vi "Global_ACT Write_Data Out.vi"() -> ()   [LabVIEW 2017, in "Lift.lvlib"]
uses:
  Lift.lvlib
  CLUSTER_ACT_Lift Output.ctl
  _SHARE ALL/RoboRio Share All/SRX Share All/TypeDefs SRX/Cluster_SRX_General Data.ctl
  _SHARE ALL/RoboRio Share All/SRX Share All/TypeDefs SRX/Cluster_SRX_Common Runtime Data.ctl
  _SHARE ALL/RoboRio Share All/SRX Share All/TypeDefs SRX/Cluster_SRX_Error Calculations.ctl
  _SHARE ALL/RoboRio Share All/SRX Share All/TypeDefs SRX/Cluster_SRX_Voltage Out Data.ctl
  _SHARE ALL/RoboRio Share All/SRX Share All/TypeDefs SRX/Cluster_SRX_Sensor Out Data.ctl
  _SHARE ALL/RoboRio Share All/SRX Share All/TypeDefs SRX/Cluster_SRX_Sensor Quad Data.ctl
  _SHARE ALL/RoboRio Share All/SRX Share All/TypeDefs SRX/Cluster_SRX_Analog In Data.ctl
  _SHARE ALL/RoboRio Share All/SRX Share All/TypeDefs SRX/Cluster_SRX_PWM Sensor Data.ctl
  _SHARE ALL/RoboRio Share All/SRX Share All/TypeDefs SRX/Cluster_SRX_F and R Limit Indicators.ctl
panel:
  in  "Lift_ACT_Rotate_Output":T1 {"Common Runtime Data Out"."Temp" format="%.1f"; "Common Runtime Data Out"."Voltage"."Bus" format="%.3f"; "Common Runtime Data Out"."Voltage"."Output" format="%.3f"; "Common Runtime Data Out"."Voltage"."Percent" format="%.3f"; "Common Runtime Data Out"."Current" format="%.2f"}
  in  "Lift_ACT_Telescope_Output":T1 {"Common Runtime Data Out"."Temp" format="%.1f"; "Common Runtime Data Out"."Voltage"."Bus" format="%.3f"; "Common Runtime Data Out"."Voltage"."Output" format="%.3f"; "Common Runtime Data Out"."Voltage"."Percent" format="%.3f"; "Common Runtime Data Out"."Current" format="%.2f"}
  in  "Lift_ACT_Claw_Rotation_Output":T1 {"Common Runtime Data Out"."Temp" format="%.1f"; "Common Runtime Data Out"."Voltage"."Bus" format="%.3f"; "Common Runtime Data Out"."Voltage"."Output" format="%.3f"; "Common Runtime Data Out"."Voltage"."Percent" format="%.3f"; "Common Runtime Data Out"."Current" format="%.2f"}
  # "The Names of the Data items in the Global Variable MUST describe who the Single Writer is\nNaming Convention of all Data Items is:   \nLib Name_Loop Name (SM or SEN or ACT)_Data Name\nExamples:\nDrive_ACT_X axis\nGameController_SEN_JoystickLeft\nHopper_SM_AgitatorSpeed"
  # "C"
  # "Units"
  # "C"
  # "Units"
  # "C"
  # "Units"
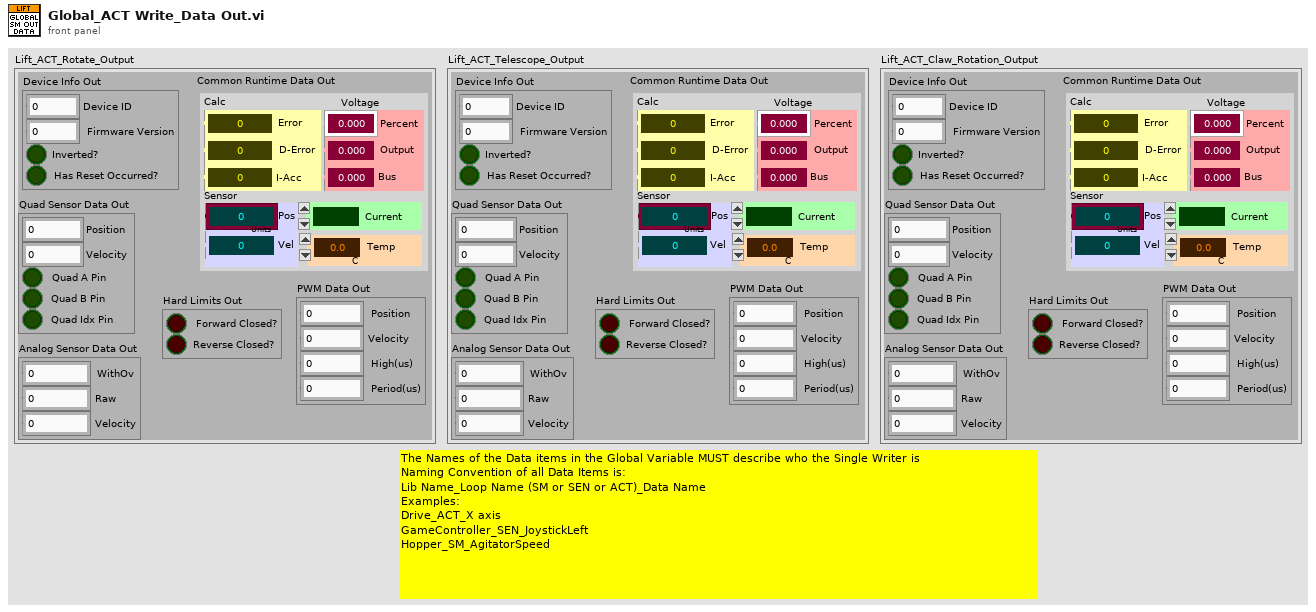
[diagram p1: front panel]
types:
  T1 = typedef "Lift.lvlib/CLUSTER_ACT_Lift Output.ctl" = cluster{"Device Info Out":T2, "Common Runtime Data Out":T3, "Quad Sensor Data Out":T7, "Analog Sensor Data Out":T8, "PWM Data Out":T9, "Hard Limits Out":T10}
  T2 = typedef "Cluster_SRX_General Data.ctl" = cluster{"Device ID":i32, "Firmware Version":i32, "Inverted?":bool, "Has Reset Occurred?":bool}
  T3 = typedef "Cluster_SRX_Common Runtime Data.ctl" = cluster{"Calc":T4, "Voltage ":T5, "Sensor":T6, "Current":dbl, "Temp":dbl}
  T4 = typedef "Cluster_SRX_Error Calculations.ctl" = cluster{"Error":i32, "D-Error":dbl, "I-Acc":dbl}
  T5 = typedef "Cluster_SRX_Voltage Out Data.ctl" = cluster{"Percent":dbl, "Output":dbl, "Bus":dbl}
  T6 = typedef "Cluster_SRX_Sensor Out Data.ctl" = cluster{"Pos":i32, "Vel":i32}
  T7 = typedef "Cluster_SRX_Sensor Quad Data.ctl" = cluster{"Position":i32, "Velocity":i32, "Quad A Pin":bool, "Quad B Pin":bool, "Quad Idx Pin":bool}
  T8 = typedef "Cluster_SRX_Analog In Data.ctl" = cluster{"WithOv":i32, "Raw":i32, "Velocity":i32}
  T9 = typedef "Cluster_SRX_PWM Sensor Data.ctl" = cluster{"Position":i32, "Velocity":i32, "High(us)":i32, "Period(us)":i32}
  T10 = typedef "Cluster_SRX_F and R Limit Indicators.ctl" = cluster{"Forward Closed?":bool, "Reverse Closed?":bool}
diagram:
